vi "Add Routing Channel.vi"(4 "description":string, 6 "initial state":string="No Connections", 8 "error in":errorcluster, 9 "state configurations":T1=[{"Name"="No Connections", "Description"="State with no connections", "Value"=-1, "Connection List"=[]}], 10 "channel name":string, 11 "routing channels in":T4 format="%.0x") -> (0 "error out":errorcluster, 2 "routing channel":T4 format="%.0x", 3 "routing channels out":T4 format="%.0x")   [LabVIEW 2020, in "Routing and Faulting Scripting.lvlib"]
doc: "Creates and adds a routing channel with the specified configuration to the custom device."
uses:
  Routing and Faulting Scripting.lvlib
  <vilib>/NI VeriStand/Custom Device API/Custom Device Item Ref.ctl
  Shared/Channel States.ctl
  Shared/Routing State.ctl
  Shared/Connection.ctl
  <vilib>/NI VeriStand/Custom Device API/Custom Device Channel.ctl
  <vilib>/NI VeriStand/Custom Device API/Custom Device Channel Type.ctl
  Shared/Constants.vi
  <vilib>/NI VeriStand/Custom Device API/Custom Device API.lvlib
  Shared/Routing and Faulting Shared.lvlib
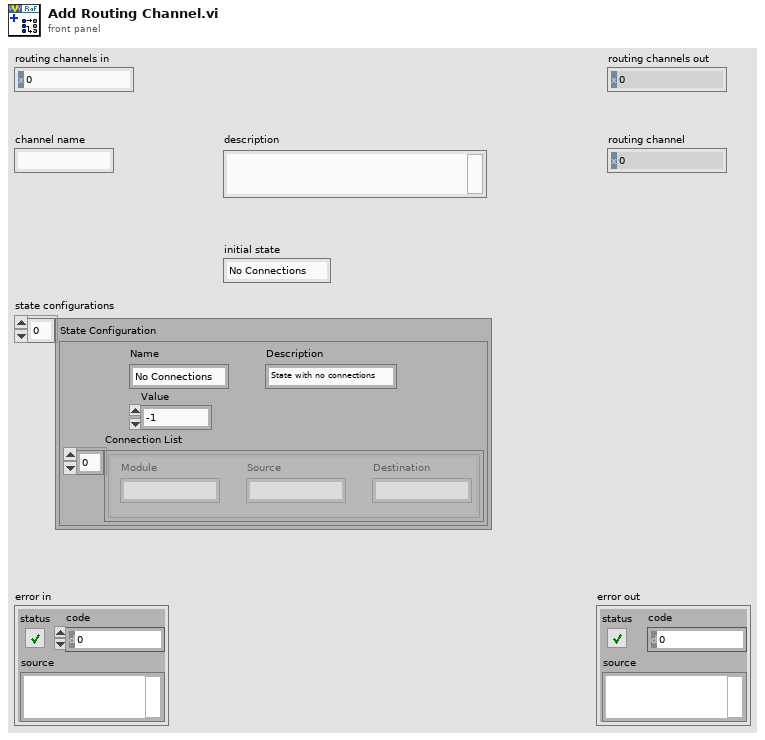
[diagram p1: front panel]
types:
  T1 = typedef "Routing and Faulting Shared.lvlib/Channel States.ctl" = T2[]
  T2 = typedef "Routing and Faulting Shared.lvlib/Routing State.ctl" = cluster{"Name":string, "Description":string, "Value":i32, "Connection List":T3[]}
  T3 = typedef "Routing and Faulting Shared.lvlib/Connection.ctl" = cluster{"Module":string, "Source":string, "Destination":string}
  T4 = typedef "Custom Device API.lvlib/Custom Device Item Ref.ctl" = u64
  T5 = typedef "Custom Device API.lvlib/Custom Device Channel.ctl" = cluster{"Type":T6, "Units":string, "Default Value":dbl, "Faultable":bool, "Scalable":bool}
  T6 = typedef "Custom Device API.lvlib/Custom Device Channel Type.ctl" = enum16{"Input", "Output"}
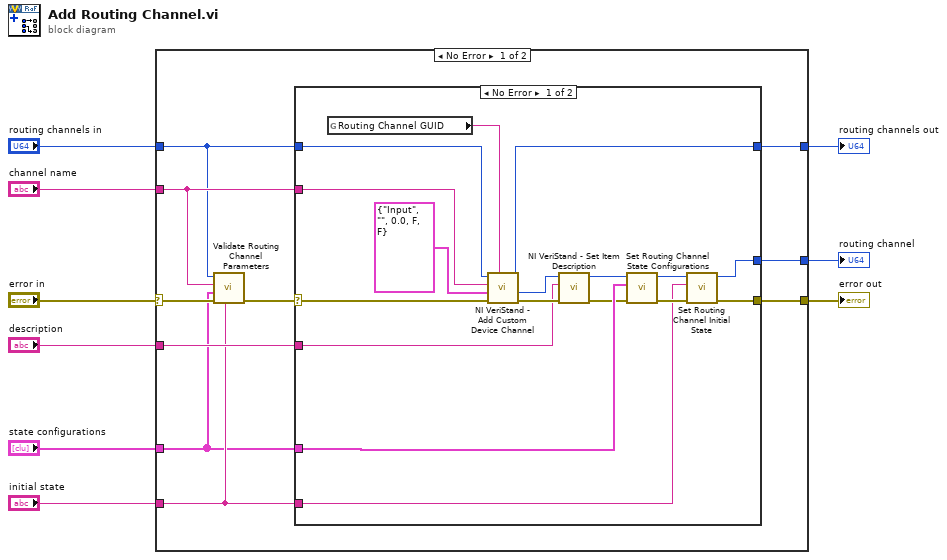
[diagram p0: block diagram]
diagram:
  n1 = case shown="No Error" "error in" {
    selector: "error in" -> [w15 w40]
    tunnel: [w17 w40] -> w9
    tunnel: [w19 w39] -> w8
    tunnel: "routing channels in" -> [w10 w39]
    tunnel: "channel name" -> [w11 _]
    tunnel: [w16 _] -> w4
    tunnel: "state configurations" -> [w12 _]
    tunnel: "description" -> [w18 _]
    tunnel: "initial state" -> [w13 _]
    frame No Error {
      n2 = call "Validate Routing Channel Parameters.vi"("initial state"=w13, "error in"=w15, "state configurations"=w12, "channel name"=w11, "routing channels in"=w10) -> ("error out"=w14:errorcluster)  [unwired: 5 in, 1 out]
      n3 = case shown="No Error" w14 {
        selector: w14 -> [w20 w37]
        tunnel: w11 -> [w36 _]
        tunnel: w12 -> [w34 _]
        tunnel: w10 -> [w33 w38]
        tunnel: [w32 w38] -> w19
        tunnel: w18 -> [w29 _]
        tunnel: [w27 w37] -> w17
        tunnel: [w25 _] -> w16
        tunnel: w13 -> [w24 _]
        frame No Error {
          n4 = global read "Constants.vi" "Routing Channel GUID"() -> (w21:string)
          n5 = call <vilib>:"NI VeriStand - Add Custom Device Channel.vi"("GUID (Default Channel)"=w21, "error in (no error)"=w20, "Channel"=T5 {"Type"=enum."Input", "Units"="", "Default Value"=0.0, "Faultable"=FALSE, "Scalable"=FALSE}, "Channel Name"=w36, "Parent Ref in"=w33) -> ("error out"=w30:errorcluster, "Channel Ref"=w28:T4, "Parent Ref out"=w32:T4)  [unwired: 3 in, 1 out]
          n6 = call <vilib>:"NI VeriStand - Set Item Description.vi"("error in (no error)"=w30, "Description"=w29, "Item Ref in"=w28) -> ("error out"=w23:errorcluster, "Item Ref out"=w22:T4)  [unwired: 6 in, 1 out]
          n7 = call "Set Routing Channel State Configurations.vi"("error in"=w23, "state configurations"=w34, "routing channel in"=w22) -> ("error out"=w35:errorcluster, "routing channel out"=w26:T4)  [unwired: 7 in]
          n8 = call "Set Routing Channel Initial State.vi"("error in"=w35, "state"=w24, "routing channel in"=w26) -> ("error out"=w27:errorcluster, "routing channel out"=w25:T4)  [unwired: 7 in]
        }
        frame Error {
        }
      }
    }
    frame Error {
    }
  }
  "error out" <- w9
  "routing channels out" <- w8
  "routing channel" <- w4
